vi "Block Problem Function and Constraints.vi"(9 "output selector":T1, 10 "data":variant, 11 "X":dbl[](array[numeric])) -> (0 "error out":errorcluster, 1 "inequality constraint function values":dbl[](array[numeric]), 2 "equality constraint function values":dbl[](array[numeric]), 3 "objective function value":dbl)   [LabVIEW 2020]
doc: "This template is the starting point for creating an objective function, equality constraint function and inequality constraint function to be passed to the Constrained Nonlinear Optimization.vi."
uses:
  <vilib>/gmath/NumericalOptimization/cno_output select.ctl
  <vilib>/gmath/NI_Gmath.lvlib
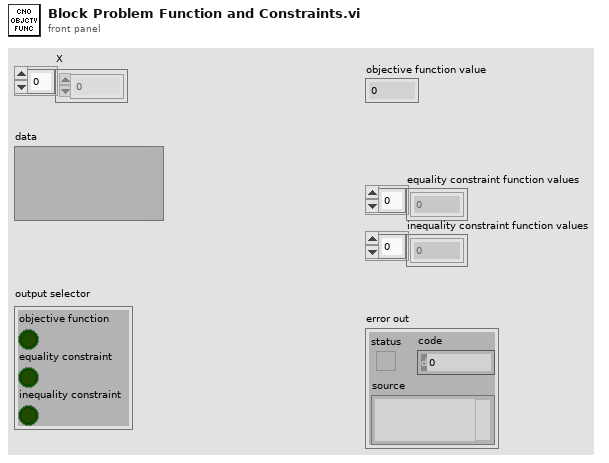
[diagram p1: front panel]
types:
  T1 = typedef "NI_Gmath.lvlib/cno_output select.ctl" = cluster{"objective function":bool, "equality constraint":bool, "inequality constraint":bool}
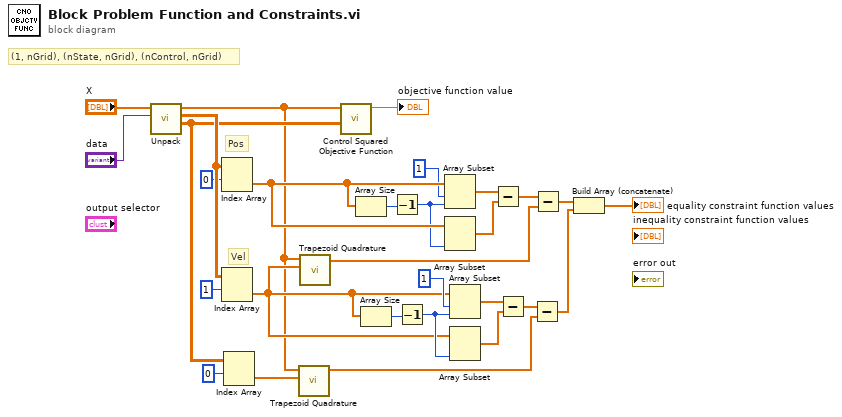
[diagram p0: block diagram]
diagram:
  # "Vel"
  # "Pos"
  # "(1, nGrid), (nState, nGrid), (nControl, nGrid)"
  n1 = call "Unpack.vi"("data"="data", "X"="X") -> ("Control"=w9:dbl[][], "State"=w26:dbl[][], "Time"=w5:dbl[])  [unwired: 7 in]
  n2 = Index Array(array=w26, index (row)=0) -> (element=w24:dbl[])  [unwired: 1 in]
  n3 = Index Array(array=w26, index (row)=1) -> (element=w13:dbl[])  [unwired: 1 in]
  n4 = Index Array(array=w9, index (row)=0) -> (element=w6:dbl[])  [unwired: 1 in]
  n5 = call "Trapezoid Quadrature.vi"("Array"=w6, "Time"=w5) -> ("Result"=w4:dbl[])  [unwired: 9 in]
  n6 = call "Trapezoid Quadrature.vi"("Array"=w13, "Time"=w5) -> ("Result"=w10:dbl[])  [unwired: 9 in]
  n7 = call "Control Squared Objective Function.vi"("Control"=w9, "Time"=w5) -> ("Objective Func"=→"objective function value":dbl)  [unwired: 9 in]
  n8 = Array Size(array=w24) -> (size(s)=w23:i32)
  n9 = Array Size(array=w13) -> (size(s)=w14:i32)
  n10 = Decrement(x=w23) -> (x-1=w22:i32)
  n11 = Decrement(x=w14) -> (x-1=w15:i32)
  n12 = Array Subset(array=w24, index=1, length=w22) -> (w21:dbl[])
  n13 = Array Subset(array=w24, length=w22) -> (w19:dbl[])  [unwired: 1 in]
  n14 = Array Subset(array=w13, index=1, length=w15) -> (w16:dbl[])
  n15 = Array Subset(array=w13, length=w15) -> (w18:dbl[])  [unwired: 1 in]
  n16 = Subtract(x=w21, y=w19) -> (x-y=w12:dbl[])
  n17 = Subtract(x=w16, y=w18) -> (x-y=w11:dbl[])
  n18 = Subtract(x=w11, y=w4) -> (x-y=w2:dbl[])
  n19 = Subtract(x=w12, y=w10) -> (x-y=w3:dbl[])
  n20 = Build Array (concatenate)(w3, w2) -> (→"equality constraint function values":dbl[])
